vi "BoxMonitor.vi"   [LabVIEW 2016]
uses:
  Instrument_Setup.vi
  <vilib>/Instr/_visa.llb/VISA Configure Serial Port (Instr).vi
  Global/Global Variables/Data_Display_global.vi
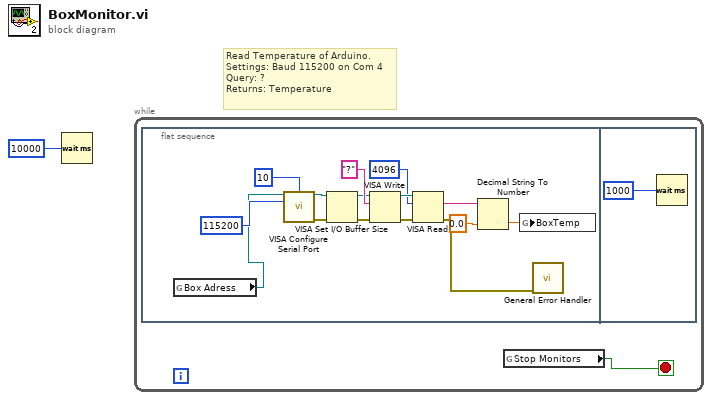
[diagram p0: block diagram]
diagram:
  # "Read Temperature of Arduino. \nSettings: Baud 115200 on Com 4\nQuery: ?\nReturns: Temperature"
  n1 = Wait (ms)(milliseconds to wait=10000) -> ()  [unwired: 1 out]
  n2 = while {
    stop <- w2 stop-if-true
    n3 = flat-sequence {
      frame #0 {
        n4 = global read "Instrument_Setup.vi" "Box Adress"() -> (w4:refnum<visa-resource-name>)
        n5 = call-poly "VISA Configure Serial Port"("VISA resource name"=w4, "termination char\n(0xA = '\\n' = LF)"=u8 10 ("termination char\n(0xA = '\\n' = LF)"), "baud rate (9600)"=115200) -> ("VISA resource name out"=w9:refnum<visa-resource-name>, "error out"=w11:errorcluster)  [unwired: 11 in]
        n6 = VISA Set I/O Buffer Size(VISA resource name=w9, error in (no error)=w11) -> (VISA resource name out=w10:refnum<visa-resource-name>, error out=w8:errorcluster)  [unwired: 2 in]
        n7 = VISA Write(VISA resource name=w10, write buffer="?", error in (no error)=w8) -> (VISA resource name out=w17:refnum<visa-resource-name>, error out=w16:errorcluster)  [unwired: 1 out]
        n8 = VISA Read(VISA resource name=w17, byte count=4096, error in (no error)=w16) -> (read buffer=w7:string, error out=w3:errorcluster)  [unwired: 2 out]
        n9 = Decimal String To Number(string=w7, default (0L)=0.0) -> (number=w5:dbl)  [unwired: 1 in, 1 out]
        n10 = global write "Data_Display_global.vi" "BoxTemp"(w5) -> ()
        n11 = call <vilib>:"General Error Handler.vi"("error in (no error)"=w3) -> ()  [unwired: 10 in, 5 out]
      }
      frame #1 {
        n12 = Wait (ms)(milliseconds to wait=1000) -> ()  [unwired: 1 out]
      }
    }
    n13 = global read "Data_Display_global.vi" "Stop Monitors"() -> (w2:bool)
  }
